vi "例11.6MSO2.vi"() -> ()   [LabVIEW 2015]
doc: "This example demonstrates how to continuously re-generate analog output data from a buffer in your computer's memory.\n\nRequires Digilent instrumentation product."
uses:
  <vilib>/Utility/error.llb/DialogType.ctl
  <vilib>/DigilentWF/DigilentWF.lvlib
panel:
  in  "Vertical Offset":dbl
  in  "Vertical Range":dbl=1.0
  in  "Device Name":string
  in  "Stop":bool
  in  "Analog Channel":string="mso/1" caption="Channel"
  out "Analog Data":waveform(dbl)[](graph)
  # "MSO Channel Settings"
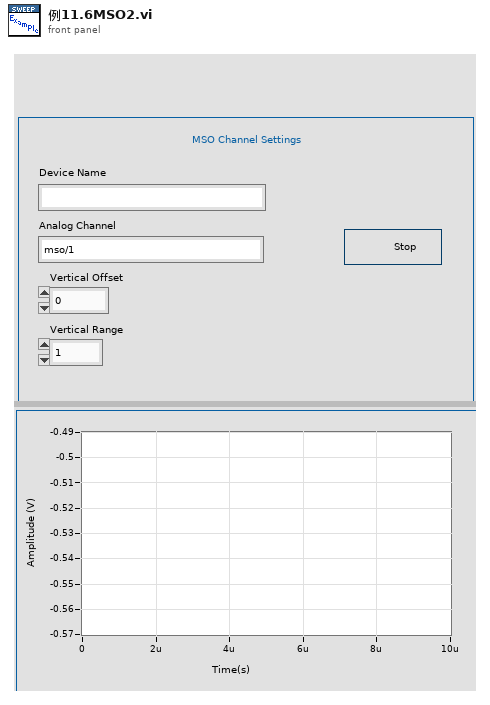
[diagram p1: front panel]
types:
  T1 = typedef "DialogType.ctl" = u16
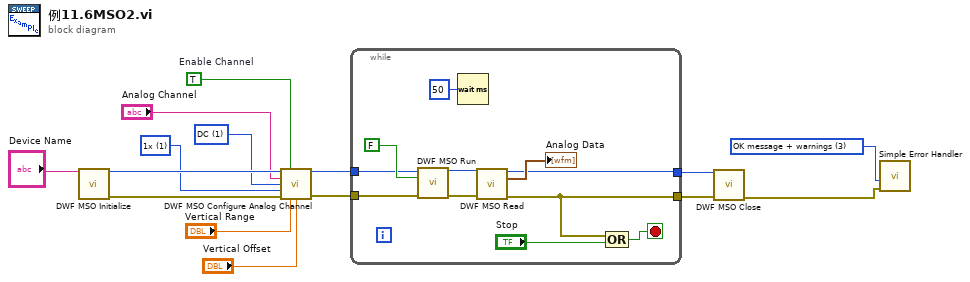
[diagram p0: block diagram]
diagram:
  w8 = 1 items=["1x"=1, "10x"=10] ("Probe Attenuation")
  w9 = 1 items=["AC", "DC"] ("Vertical Coupling")
  w1 = TRUE  # Enable Channel
  w15 = T1 3 items=["no dialog", "OK message", "continue or stop message", "OK message + warnings", "continue/stop + warnings"] ("type of dialog (OK msg:1)")
  n1 = call <vilib>:"DWF MSO Initialize.vi"("Device Name"="Device Name") -> ("Instrument Handle Out"=w13:u32, "Error Out"=w14:errorcluster)  [unwired: 13 in]
  n2 = call <vilib>:"DWF MSO Configure Analog Channel.vi"("Instrument Handle In"=w13, "Enable Channel"=w1, "Channel"="Analog Channel", "Vertical Coupling"=w9, "Probe Attenuation"=w8, "Error In"=w14, "Vertical Range"="Vertical Range", "Vertical Offset"="Vertical Offset") -> ("Instrument Handle Out"=w3:u32, "Error Out"=w2:errorcluster)  [unwired: 6 in]
  n3 = while {
    tunnel: [w25] -> w12
    tunnel: [w22] -> w11
    tunnel: w3 -> [w17]
    tunnel: w2 -> [w16]
    stop <- w24 stop-if-true
    n4 = call <vilib>:"DWF MSO Run.vi"("Instrument Handle In"=w17, "Auto Trigger"=FALSE, "Error In"=w16) -> ("Instrument Handle Out"=w21:u32, "Error Out"=w20:errorcluster)  [unwired: 11 in]
    n5 = Wait (ms)(milliseconds to wait=u32 50) -> ()  [unwired: 1 out]
    n6 = call <vilib>:"DWF MSO Read.vi"("Instrument Handle In"=w21, "Error In"=w20) -> ("Instrument Handle Out"=w22:u32, "Analog Waveforms"=→"Analog Data":waveform(dbl)[], "Error Out"=w25:errorcluster)  [unwired: 8 in, 3 out]
    n7 = Compound Arithmetic op=OR(w25, "Stop") -> (w24:bool)
  }
  n8 = call <vilib>:"DWF MSO Close.vi"("Instrument Handle In"=w11, "Error In"=w12) -> ("Error Out"=w6:errorcluster)  [unwired: 13 in]
  n9 = call <vilib>:"Simple Error Handler.vi"("type of dialog (OK msg:1)"=w15, "error in (no error)"=w6) -> ()  [unwired: 3 in, 5 out]
